vi "Controller - State Process.vi"(8 "error in (no error)":errorcluster, 11 "View Model":T1) -> (0 "error out":errorcluster, 3 "View Model":T1)   [LabVIEW 2017]
doc: "Orginize state transition and process current state"
uses:
  View Model/Controls/View Model.ctl
  Error Handler/Controls/Error Model.ctl
  Error Handler/Controls/Error Data.ctl
  Error Handler/Controls/Error Type.ctl
  View Model/Controls/Shared Model.ctl
  Configuration/Controls/Config Model.ctl
  Configuration/Controls/Config CMD.ctl
  Configuration/Controls/Config Data.ctl
  Controls/Controller Model.ctl
  Controls/Controller Overhead.ctl
  Controls/Controller States.ctl
  Controls/Controller Message Data.ctl
  Controls/Controller Message Name.ctl
  Views/User Console View/Controls/User Console - Keypad.ctl
  Views/User Console View/Controls/User Console - Transactions.ctl
  Controls/Controller CMD.ctl
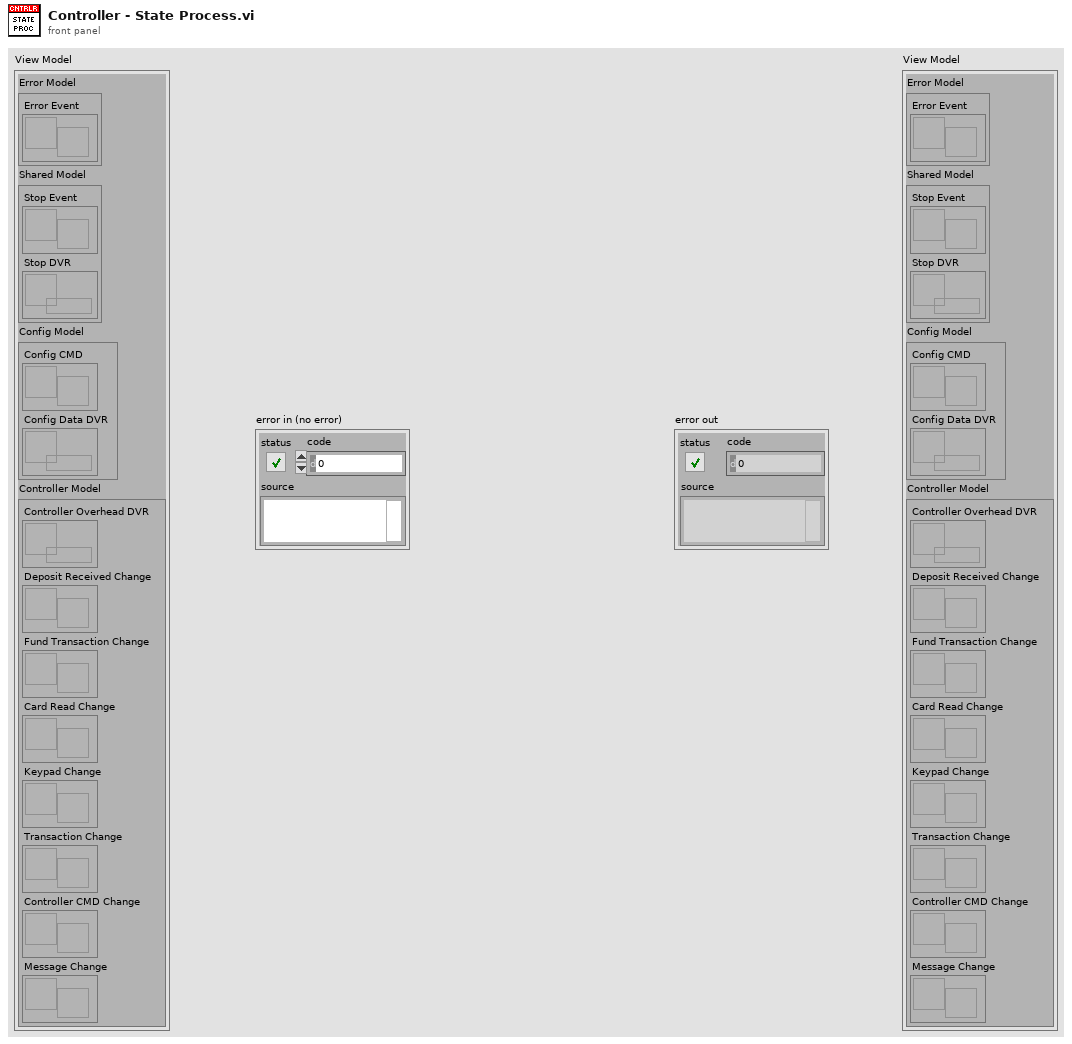
[diagram p1: front panel]
types:
  T1 = typedef "View Model.ctl" = cluster{"Error Model":T2, "Shared Model":T3, "Config Model":T4, "Controller Model":T5}
  T2 = typedef "Error Model.ctl" = cluster{"Error Event":refnum<user-event>}
  T3 = typedef "Shared Model.ctl" = cluster{"Stop Event":refnum<user-event>, "Stop DVR":refnum<data-value>}
  T4 = typedef "Config Model.ctl" = cluster{"Config CMD":refnum<user-event>, "Config Data DVR":refnum<data-value>}
  T5 = typedef "Controller Model.ctl" = cluster{"Controller Overhead DVR":refnum<data-value>, "Deposit Received Change":refnum<user-event>, "Fund Transaction Change":refnum<user-event>, "Card Read Change":refnum<user-event>, "Keypad Change":refnum<user-event>, "Transaction Change":refnum<user-event>, "Controller CMD Change":refnum<user-event>, "Message Change":refnum<user-event>}
  T6 = typedef "Controller States.ctl" = enum16{"Idle", "Init", "Display Message", "Login", "Balance Inquiry", "Deposit", "Withdrawal", "Fast Cash", "Terminate"}
  T7 = typedef "Controller Message Name.ctl" = enum16{"Welcome", "Login", "Idle", "Invalid Login", "Terminate", "Deposit", "Withdrawal", "Fast Cash", "Withdrawal Complete", "Withdrawal Failed", "Balance Inquiry"}
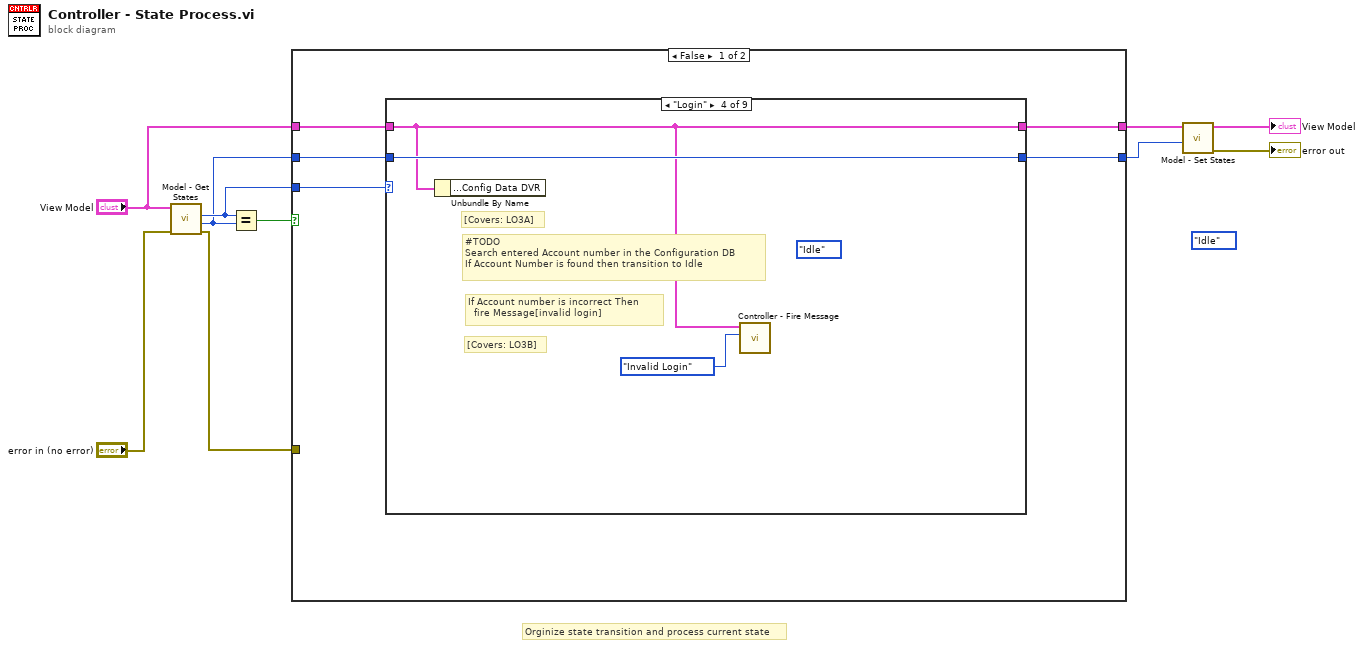
[diagram p0: block diagram]
diagram:
  (unwired) Controller_States."Idle" ("Current State")
  # "Orginize state transition and process current state"
  n1 = call "Model - Get States.vi"("error in (no error)"="error in (no error)", "View Model"="View Model") -> ("error out"=w6:errorcluster, "Next State"=w8:T6, "Current State"=w9:T6)  [unwired: 6 in, 1 out]
  n2 = Equal?(x=w9, y=w8) -> (x = y?=w10:bool)
  n3 = case shown="False" w10 {
    tunnel: w9 -> [w15 _]
    tunnel: w8 -> [w14 w35]
    tunnel: w6 -> [_ _]
    tunnel: [w13 w35] -> w3
    tunnel: "View Model" -> [w12 _]
    tunnel: [w11 _] -> w4
    frame False {
      n4 = case shown="\"Login\"" w15 {
        tunnel: w14 -> [w17 w19 w21 w24 w26 w28 w30 w32 w34]
        tunnel: [w17 w19 w21 w24 w26 w28 w30 w32 w34] -> w13
        tunnel: w12 -> [w16 w18 w20 w23 w25 w27 w29 w31 w33]
        tunnel: [w16 w18 w20 w23 w25 w27 w29 w31 w33] -> w11
        frame "Idle", Default {
        }
        frame "Init" {
        }
        frame "Display Message" {
        }
        frame "Login" {
          (unwired) Controller_States."Idle" ("Current State")
          # "[Covers: LO3B]"
          # "If Account number is incorrect Then \n  fire Message[invalid login]"
          # "[Covers: LO3A]"
          # "#TODO\nSearch entered Account number in the Configuration DB\nIf Account Number is found then transition to Idle"
          n5 = Unbundle By Name(w23) -> ()  [unwired: 1 out]
          n6 = call "Controller - Fire Message.vi"("Message Name"=Controller_Message_Name."Invalid Login", "View Model"=w23) -> ()  [unwired: 8 in, 2 out]
        }
        frame "Balance Inquiry" {
        }
        frame "Deposit" {
        }
        frame "Withdrawal" {
        }
        frame "Fast Cash" {
        }
        frame "Terminate" {
        }
      }
    }
    frame True {
    }
  }
  n7 = call "Model - Set States.vi"("Next State"=w3, "View Model"=w4) -> ("error out"=→"error out":errorcluster, "View Model"=→"View Model":T1)  [unwired: 8 in]
